vi "Query Number of Periods.vi"(8 "error in (no error)":errorcluster, 11 "VISA resource name":refnum<visa-resource-name>) -> (0 "error out":errorcluster, 2 "output":dbl, 3 "VISA resource name out":refnum<visa-resource-name>)   [LabVIEW 2009, in "SR400.lvlib"]
doc: "NP { m }\nIf m is absent, the NP command returns the\nprogrammed number of periods in a scan (N\nPERIODS). If m is included, the number of\nperiods is set to the value m. The parameter m\nmust be an integer from 1 to 2000. Changing the\nnumber of periods during a scan is allowed. If the\nnew value exceeds the current scan position, then\nthe scan will continue to the new number of\nperiods. If the new value is lower than the current\nscan position, then the scan ends at the next end of\ncount period."
uses:
  SR400.lvlib
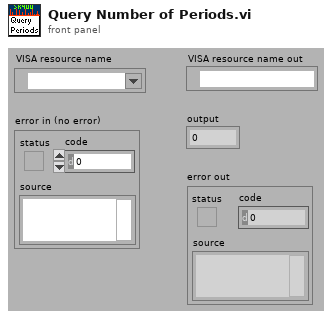
[diagram p1: front panel]
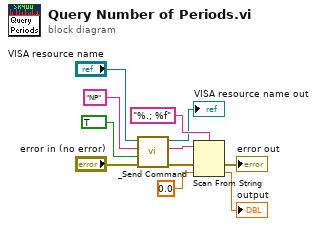
[diagram p0: block diagram]
diagram:
  n1 = call "_Send Command.vi"("error in (no error)"="error in (no error)", "Query? (F)"=TRUE, "Command"="NP" ("command"), "VISA resource name"="VISA resource name") -> ("error out"=w2:errorcluster, "Response"=w3:string, "VISA resource name out"=→"VISA resource name out":refnum<visa-resource-name>)  [unwired: 5 out]
  n2 = Scan From String(format string="%.; %f", input string=w3, error in=w2, default 1=0.0 ("default value 1")) -> (error out=→"error out":errorcluster, output 1=→"output":dbl)  [unwired: 1 in, 2 out]
